vi "ST example routine.vi"() -> ()   [LabVIEW 2009]
panel:
  out "Motor Speed\nSteps/sec":string
  out "Changed speed":bool
  out "MOTORS OFF\nDONE":bool
  out "STATUS\nREADY":bool
  out "Performed\nWAIST -0.4 radians":bool
  out "Proformed\nWAIST 0.4 radians":bool
  # "THIS IS A TEST ROUTINE FOR THE MOTIONS\nFIRST IT WILL INITIALIZE THE ROBOT AND THE CONTROLLER\nTHEN IT WILL EXERCISE A JOINT\nCHANGING SPEED BETWEEN MOVES\nIT THEN WILL DE-ENERGIZE THE MOTORS."
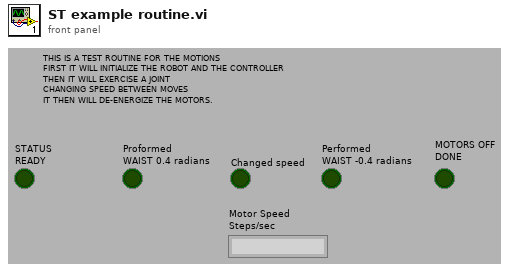
[diagram p1: front panel]
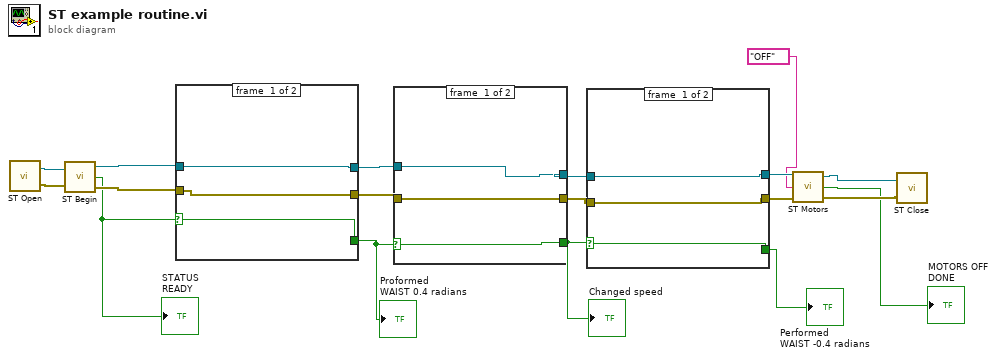
[diagram p0: block diagram]
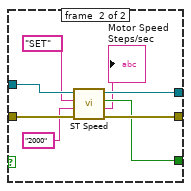
[diagram p2: hidden frame]
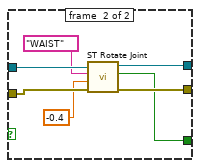
[diagram p3: hidden frame]
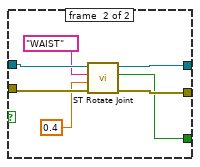
[diagram p4: hidden frame]
diagram:
  n1 = call "ST Open.vi"() -> ("VISA resource name out"=w17:refnum<visa-resource-name>, "error out"=w16:errorcluster)  [unwired: 1 in]
  n2 = call "ST Begin.vi"("VISA resource name in"=w17, "error in"=w16) -> ("VISA resource name out"=w15:refnum<visa-resource-name>, "Begin Complete"=w13:bool, "error out"=w14:errorcluster)
  "STATUS\nREADY" <- w13
  n3 = case shown="True" w13 {
    selector: w13 -> [w19 _]
    tunnel: w15 -> [w21 w28]
    tunnel: w14 -> [w20 w27]
    tunnel: [w21 w25] -> w6
    tunnel: [w20 w24] -> w5
    tunnel: [w19 w23] -> w2
    frame #0 {
    }
    frame #1 {
      n4 = call "ST Rotate Joint.vi"("error in (no error)"=w27, "Radians"=0.4, "Joint to rotate"="WAIST" ("JOINT NAME"), "VISA resource name"=w28) -> ("error out"=w24:errorcluster, "Ready and OK"=w23:bool, "VISA resource name out"=w25:refnum<visa-resource-name>)  [unwired: 2 out]
    }
  }
  "Proformed\nWAIST 0.4 radians" <- w2
  n5 = case shown="True" w2 {
    selector: w2 -> [w29 _]
    tunnel: w6 -> [w31 w39]
    tunnel: w5 -> [w30 w38]
    tunnel: [w30 w37] -> w4
    tunnel: [w31 w36] -> w3
    tunnel: [w29 w33] -> w1
    frame #0 {
    }
    frame #1 {
      n6 = call "ST Speed.vi"("error in (error out)"=w38, "New Speed"="2000", "Action"="SET", "VISA resource name in"=w39) -> ("error out"=w37:errorcluster, "Motor Speed"=→"Motor Speed\nSteps/sec":string, "Complete"=w33:bool, "VISA resource name out"=w36:refnum<visa-resource-name>)
    }
  }
  "Changed speed" <- w1
  n7 = case shown="True" w1 {
    selector: w1 -> [w40 _]
    tunnel: w3 -> [w42 w49]
    tunnel: w4 -> [w41 w48]
    tunnel: [w42 w46] -> w11
    tunnel: [w41 w45] -> w12
    tunnel: [w40 w44] -> w18
    frame #0 {
    }
    frame #1 {
      n8 = call "ST Rotate Joint.vi"("error in (no error)"=w48, "Radians"=-0.4, "Joint to rotate"="WAIST" ("JOINT NAME"), "VISA resource name"=w49) -> ("error out"=w45:errorcluster, "Ready and OK"=w44:bool, "VISA resource name out"=w46:refnum<visa-resource-name>)  [unwired: 2 out]
    }
  }
  "Performed\nWAIST -0.4 radians" <- w18
  n9 = call "ST Motors.vi"("error in (error out)"=w12, "Combo Box"="OFF", "VISA resource name in"=w11) -> ("error out"=w9:errorcluster, "SESSION \nENDED"=→"MOTORS OFF\nDONE":bool, "VISA resource name out"=w10:refnum<visa-resource-name>)
  n10 = call "ST Close.vi"("error in (no error)"=w9, "VISA resource name"=w10) -> ()
